vi "Day 10 Puzzle 1.vi"(11 "Path":path) -> ()   [LabVIEW 2021]
uses:
  <vilib>/Utility/file.llb/Read Delimited Spreadsheet (string).vi
panel:
  out "sum":i32
  out "Array 2":i32[](array[numeric])
  out "Array":cluster{"Cycle Number":i32, "X":i32}[](array[cluster])
  out "Cluster":cluster{"Cycle Number":i32, "X":i32}
  out "subarray":string[](array[string])
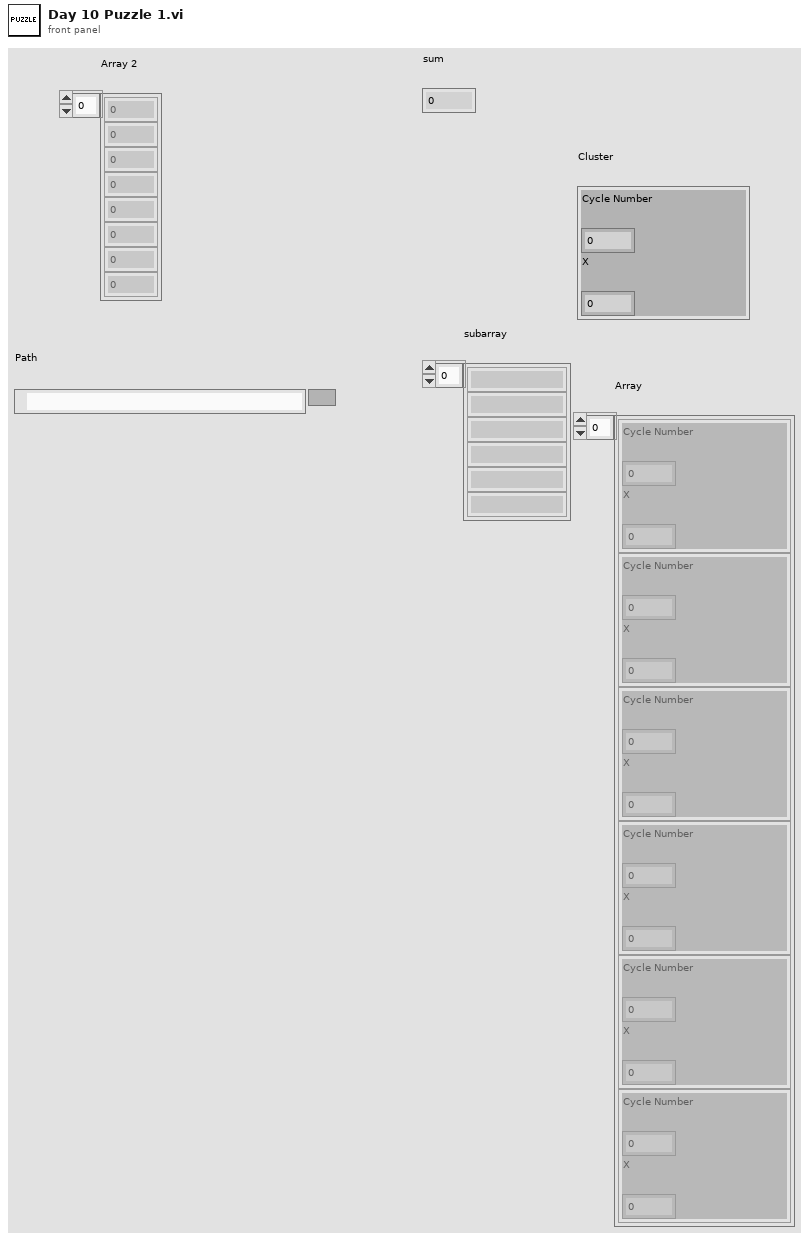
[diagram p1: front panel]
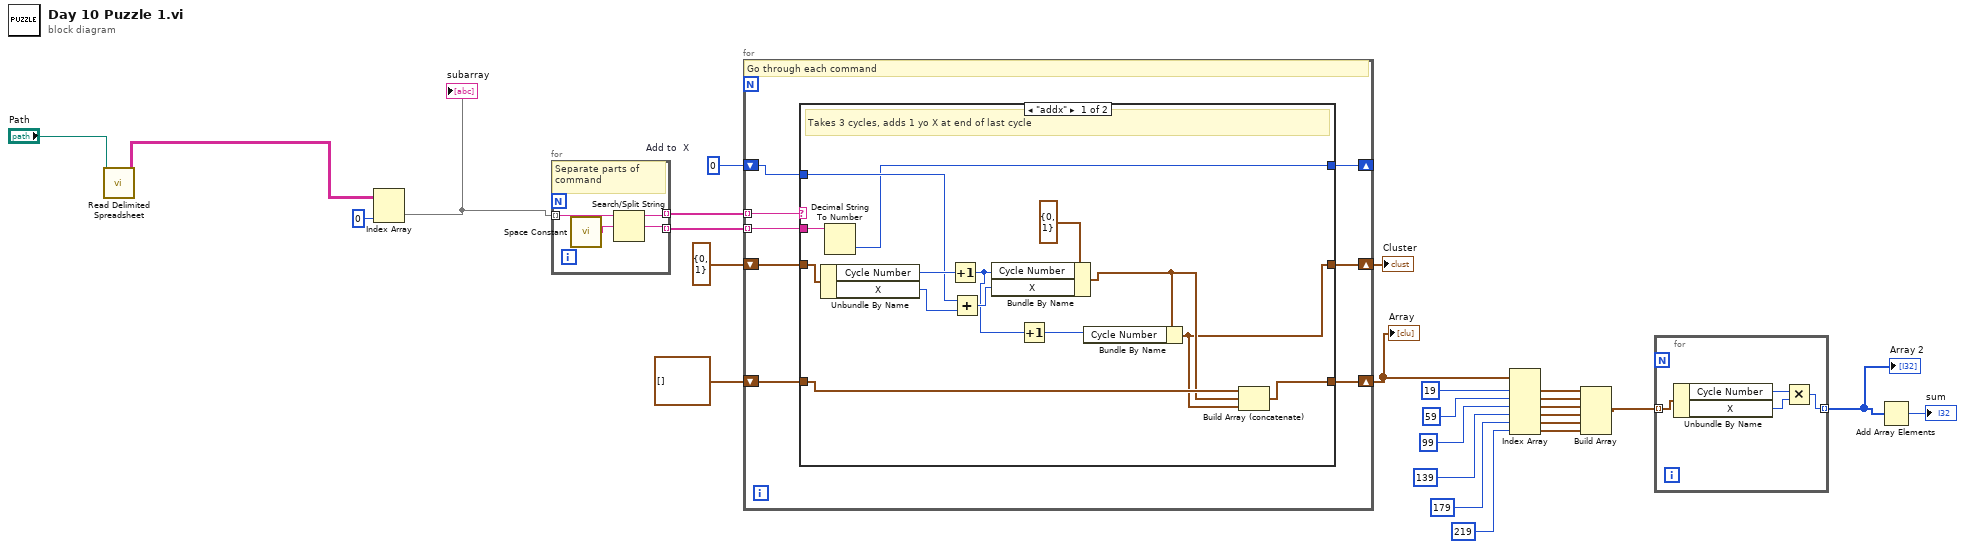
[diagram p0: block diagram]
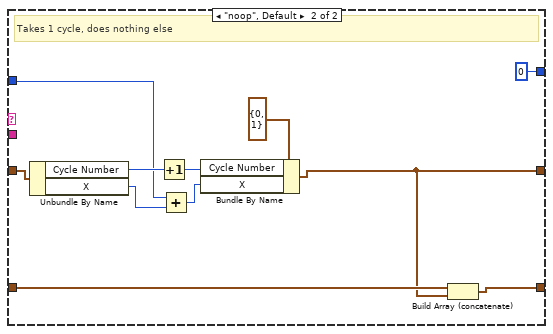
[diagram p2: hidden frame]
diagram:
  w17 = 0  # Add to  X
  n1 = call-poly <vilib>:"Read Delimited Spreadsheet.vi"("file path (dialog if empty)"="Path") -> ("all rows"=w25:string[][])  [unwired: 9 in, 5 out]
  n2 = Index Array(array=w25, index (col)=0 ("disabled index (col)")) -> (element=w23:string[])  [unwired: 1 in]
  "subarray" <- w23
  n3 = for {
    tunnel: w23 -> [w30] mode=indexing
    tunnel: [w28] -> w22 mode=indexing
    tunnel: [w27] -> w21 mode=indexing
    # "Separate parts of command"
    n4 = call <vilib>:"Space Constant.vi"() -> ("String"=w29:string)
    n5 = Search/Split String(string=w30, search string/char (-)=w29) -> (substring before match=w28:string, match + rest of string=w27:string)  [unwired: 1 in, 1 out]
  }
  n6 = for {
    tunnel: w22 -> [w38] mode=indexing
    tunnel: w21 -> [w37] mode=indexing
    shift-right: [w33] -> w16
    shift-left: cluster{"Cycle Number":i32, "X":i32}[] [] -> [w36]
    shift-right: [w34] -> w18
    shift-left: cluster{"Cycle Number":i32, "X":i32} {"Cycle Number"=0, "X"=1} ("Cluster") -> [w35]
    shift-right: [w31] -> _
    shift-left: w17 -> [w32]
    # "Go through each command"
    n7 = case shown="\"addx\"" w38 {
      tunnel: w37 -> [w42 _]
      tunnel: w36 -> [w48 w57]
      tunnel: w35 -> [w43 w62]
      tunnel: [w39 w56] -> w34
      tunnel: [w47 w55] -> w33
      tunnel: w32 -> [w41 w53]
      tunnel: [w40 0] -> w31
      frame "addx" {
        # "Takes 3 cycles, adds 1 yo X at end of last cycle"
        n8 = Unbundle By Name(w43) -> ("Cycle Number"=w51:i32, "X"=w50:i32)
        n9 = Decimal String To Number(string=w42) -> (number=w40:i32)  [unwired: 2 in, 1 out]
        n10 = Increment(x=w51) -> (x+1=w45:i32)
        n11 = Add(x=w41, y=w50) -> (x+y=w49:i32)
        n12 = Bundle By Name(cluster=cluster{"Cycle Number":i32, "X":i32} {"Cycle Number"=0, "X"=1} ("Cluster"), "Cycle Number"=w45, "X"=w49) -> (w46:cluster{"Cycle Number":i32, "X":i32})
        n13 = Increment(x=w45) -> (x+1=w44:i32)
        n14 = Bundle By Name(cluster=w46, "Cycle Number"=w44) -> (w39:cluster{"Cycle Number":i32, "X":i32})
        n15 = Build Array (concatenate)(w48, w46, w39) -> (w47:cluster{"Cycle Number":i32, "X":i32}[])
      }
      frame "noop", Default {
        # "Takes 1 cycle, does nothing else"
        n16 = Unbundle By Name(w62) -> ("Cycle Number"=w61:i32, "X"=w59:i32)
        n17 = Increment(x=w61) -> (x+1=w60:i32)
        n18 = Add(x=w53, y=w59) -> (x+y=w58:i32)
        n19 = Bundle By Name(cluster=cluster{"Cycle Number":i32, "X":i32} {"Cycle Number"=0, "X"=1} ("Cluster"), "Cycle Number"=w60, "X"=w58) -> (w56:cluster{"Cycle Number":i32, "X":i32})
        n20 = Build Array (concatenate)(w57, w56) -> (w55:cluster{"Cycle Number":i32, "X":i32}[])
      }
    }
  }
  "Cluster" <- w18
  "Array" <- w16
  n21 = Index Array(array=w16, index #1=19 ("index"), index #2=59 ("index"), index #3=99 ("index"), index #4=139 ("index"), index #5=179 ("index"), index #6=219 ("index")) -> (element #1=w9:cluster{"Cycle Number":i32, "X":i32}, element #2=w8:cluster{"Cycle Number":i32, "X":i32}, element #3=w7:cluster{"Cycle Number":i32, "X":i32}, element #4=w6:cluster{"Cycle Number":i32, "X":i32}, element #5=w5:cluster{"Cycle Number":i32, "X":i32}, element #6=w4:cluster{"Cycle Number":i32, "X":i32})
  n22 = Build Array(w9, w8, w7, w6, w5, w4) -> (w3:cluster{"Cycle Number":i32, "X":i32}[])
  n23 = for {
    tunnel: w3 -> [w67] mode=indexing
    tunnel: [w64] -> w2 mode=indexing
    n24 = Unbundle By Name(w67) -> ("Cycle Number"=w66:i32, "X"=w65:i32)
    n25 = Multiply(x=w66, y=w65) -> (x*y=w64:i32)
  }
  "Array 2" <- w2
  n26 = Add Array Elements(numeric array=w2) -> (sum=→"sum":i32)
